vi "SynapseAPI-Delete Block.vi"(0 "URL":string="http://localhost:24414", 7 "block":string, 11 "error in (no error)":errorcluster) -> (15 "error out":errorcluster)   [LabVIEW 2020]
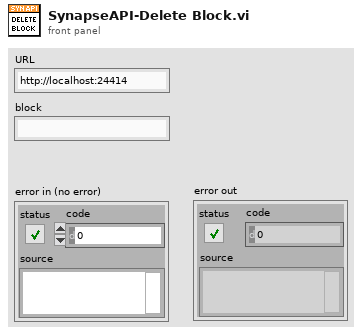
[diagram p1: front panel]
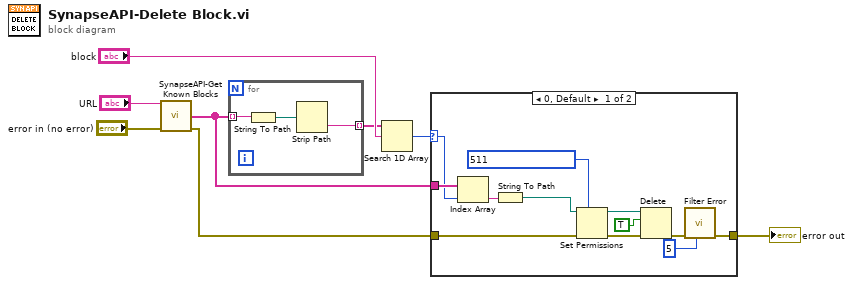
[diagram p0: block diagram]
diagram:
  n1 = call "SynapseAPI-Get Known Blocks.vi"("URL"="URL", "error in (no error)"="error in (no error)") -> ("blocks"=w5:string[], "error out"=w2:errorcluster)  [unwired: 12 in]
  n2 = for {
    tunnel: w5 -> [w11] mode=indexing
    tunnel: [w9] -> w1 mode=indexing
    n3 = String To Path(string=w11) -> (path=w10:path)
    n4 = Strip Path(path=w10) -> (name=w9:string)  [unwired: 1 out]
  }
  n5 = Search 1D Array(1D array=w1, element="block") -> (index of element=w4:i32)  [unwired: 1 in]
  n6 = case shown="0, Default" w4 {
    selector: w4 -> [w22 _]
    tunnel: w5 -> [w23 _]
    tunnel: w2 -> [w17 w24]
    tunnel: [w13 w24] -> w3
    frame 0, Default {
      n7 = Index Array(array=w23, index=w22) -> (element=w20:string)
      n8 = String To Path(string=w20) -> (path=w16:path)
      n9 = Set Permissions(7:i16 511 ("permissions"), 8:w17, 11:w16) -> (0:w18:errorcluster, 3:w15:path)  [unwired: 2 in]
      n10 = Delete(path (use dialog)=w15, entire hierarchy (F)=TRUE, error in=w18) -> (error out=w19:errorcluster)  [unwired: 2 in, 2 out]
      n11 = call "Filter Error.vi"("error in (no error)"=w19, "code to ignore"=5) -> ("error out"=w13:errorcluster)  [unwired: 9 in]
    }
    frame -1 {
    }
  }
  "error out" <- w3
